vi "Insert_subvi_to_subpanel.vi"(5 "SubVI path":path, 6 "HART resource name":refnum<visa-resource-name>="HART", 7 "subpanel ref":refnum<vi>, 8 "Input number":i32, 9 "MODBUS resource name":refnum<visa-resource-name>="485", 10 "Index":u16(ring) items=["None", "Pulse Input", "Current Input", "Serial Input"], 11 "Array of VIs to insert":string[](array[string])) -> (0 "error out":errorcluster, 3 "VI reference out":refnum<vi>)   [LabVIEW 2016]
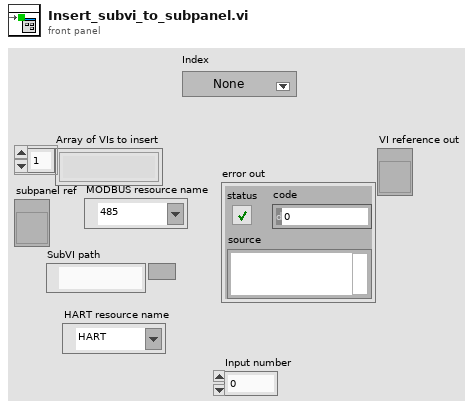
[diagram p1: front panel]
types:
  T1 = cluster{"Current Path":path, "DataFiles Path":path, "ReportFiles Path":path, "SupportFiles Path":path, "ReportTemplate Path":path, "Sample_pulses_VIT_Path":path, "Sample_current_VIT_Path":path, "Sample_MODBUS_VIT_Path":path}
  T2 = enum16{"Always On", "Always Off", "Off While Running"}
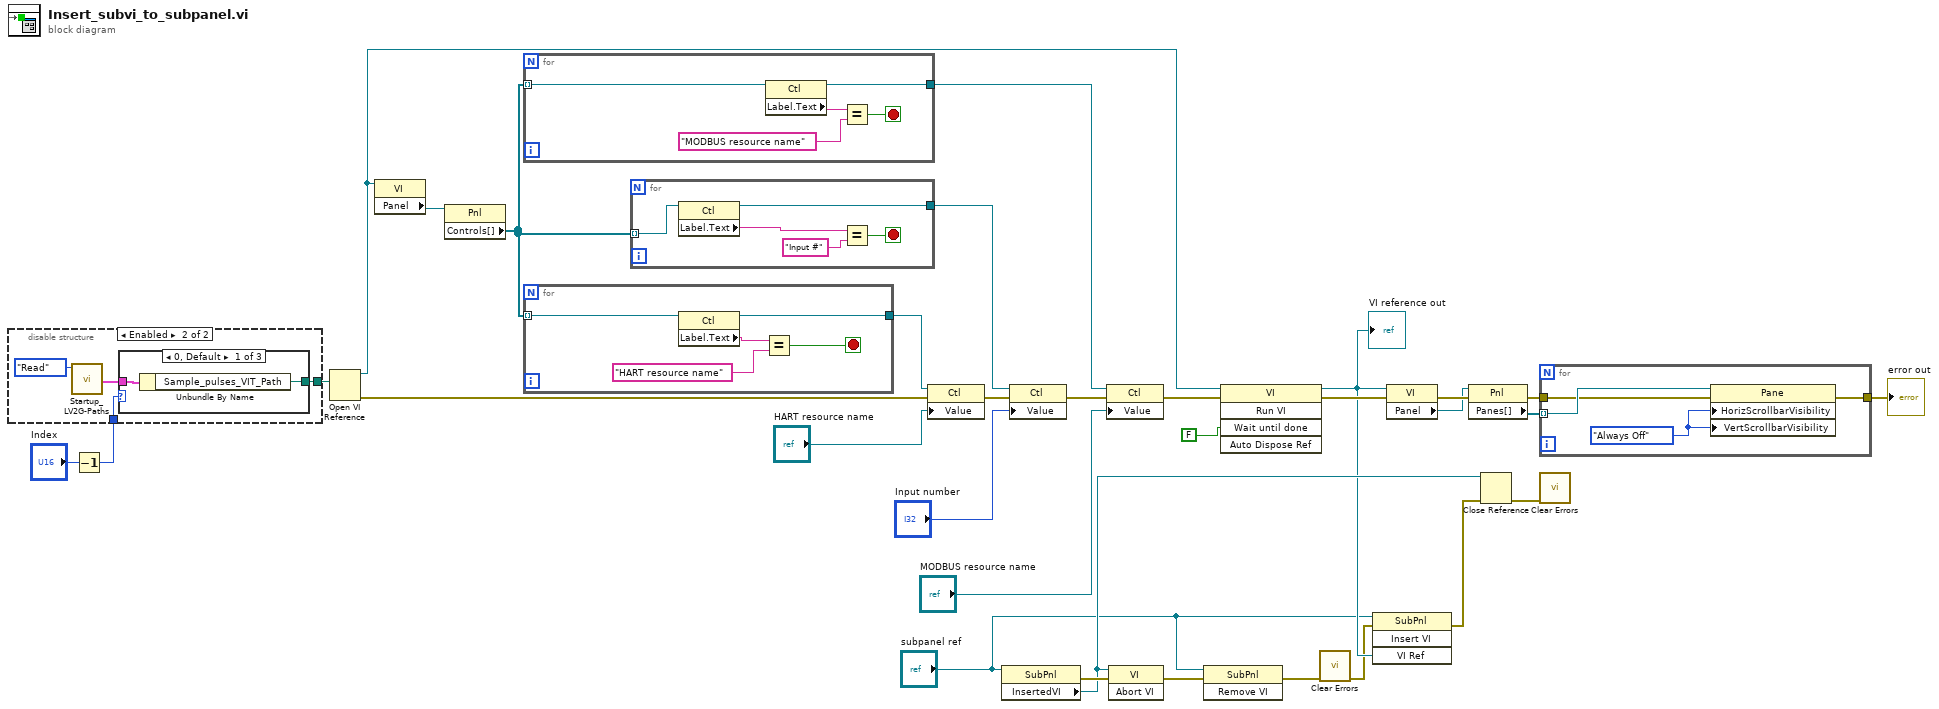
[diagram p0: block diagram]
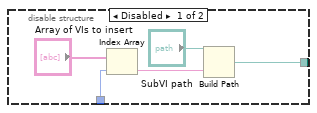
[diagram p2: hidden frame]
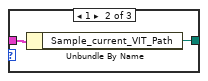
[diagram p3: hidden frame]
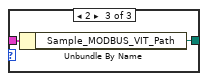
[diagram p4: hidden frame]
diagram:
  n1 = Decrement(x="Index") -> (x-1=w23:u16)
  n2 = disable-structure shown="Enabled" {
    disable-tunnel: [w37 w38] -> w30
    disable-tunnel: w23 -> [w35 w39]
    frame Disabled {
      n3 = Index Array(array="Array of VIs to insert", index=w35) -> (element=w36:string)
      n4 = Build Path(base path="SubVI path", name or relative path=w36) -> (appended path=w37:path)
    }
    frame Enabled {
      n5 = call "Startup_LV2G-Paths.vi"("Action"=enum16{"Read", "Write"}."Read") -> ("Paths"=w41:T1)  [unwired: 9 in, 1 out]
      n6 = case shown="0, Default" w39 {
        tunnel: w41 -> [w43 w45 w47]
        tunnel: [w42 w44 w46] -> w38
        frame 0, Default {
          n7 = Unbundle By Name(w43) -> ("Sample_pulses_VIT_Path"=w42:path)
        }
        frame 1 {
          n8 = Unbundle By Name(w45) -> ("Sample_current_VIT_Path"=w44:path)
        }
        frame 2 {
          n9 = Unbundle By Name(w47) -> ("Sample_MODBUS_VIT_Path"=w46:path)
        }
      }
    }
  }
  n10 = Open VI Reference(vi path=w30) -> (vi reference=w14:refnum<vi>, error out=w6:errorcluster)  [unwired: 5 in]
  n11 = property class="VI"(reference=w14) -> ("Panel"=w16:refnum<vi>)  [unwired: 1 in, 2 out]
  n12 = property class="Pnl"(reference=w16) -> ("Controls[]"=w4:refnum<vi>[])  [unwired: 1 in, 2 out]
  n13 = for {
    tunnel: w4 -> [w48] mode=indexing
    tunnel: [w49] -> w17
    stop <- w50 stop-if-true
    n14 = property class="Ctl"(reference=w48) -> (reference out=w49:refnum<vi>, "Label.Text"=w52:string)  [unwired: 1 in, 1 out]
    n15 = Equal?(x=w52, y="MODBUS resource name") -> (x = y?=w50:bool)
  }
  n16 = for {
    tunnel: w4 -> [w53] mode=indexing
    tunnel: [w54] -> w8
    stop <- w55 stop-if-true
    n17 = property class="Ctl"(reference=w53) -> (reference out=w54:refnum<vi>, "Label.Text"=w57:string)  [unwired: 1 in, 1 out]
    n18 = Equal?(x=w57, y="HART resource name") -> (x = y?=w55:bool)
  }
  n19 = for {
    tunnel: w4 -> [w58] mode=indexing
    tunnel: [w59] -> w5
    stop <- w60 stop-if-true
    n20 = property class="Ctl"(reference=w58) -> (reference out=w59:refnum<vi>, "Label.Text"=w62:string)  [unwired: 1 in, 1 out]
    n21 = Equal?(x=w62, y="Input #") -> (x = y?=w60:bool)
  }
  n22 = property class="Ctl"(reference=w8, error in=w6, "Value"="HART resource name") -> (error out=w3:errorcluster)  [unwired: 1 out]
  n23 = property class="SubPnl"(reference="subpanel ref") -> (error out=w29:errorcluster, "InsertedVI"=w27:refnum<vi>)  [unwired: 1 in, 1 out]
  n24 = property class="Ctl"(reference=w5, error in=w3, "Value"="Input number") -> (error out=w2:errorcluster)  [unwired: 1 out]
  n25 = property class="Ctl"(reference=w17, error in=w2, "Value"="MODBUS resource name") -> (error out=w15:errorcluster)  [unwired: 1 out]
  n26 = invoke class="VI" method="Abort VI"(reference=w27, error in=w29) -> (error out=w26:errorcluster)  [unwired: 1 in, 2 out]
  n27 = invoke class="SubPnl" method="Remove VI"(reference="subpanel ref", error in=w26) -> (error out=w25:errorcluster)  [unwired: 1 in, 2 out]
  n28 = invoke class="VI" method="Run VI"(reference=w14, error in=w15, "Wait until done"=FALSE ("Wait Until Done")) -> (reference out=w18:refnum<vi>, error out=w22:errorcluster)  [unwired: 2 in, 3 out]
  "VI reference out" <- w18
  n29 = call <vilib>:"Clear Errors.vi"("error in (no error)"=w25) -> ("error out"=w13:errorcluster)  [unwired: 5 in, 1 out]
  n30 = invoke class="SubPnl" method="Insert VI"(reference="subpanel ref", error in=w13, "VI Ref"=w18) -> (error out=w28:errorcluster)  [unwired: 1 in, 3 out]
  n31 = property class="VI"(reference=w18, error in=w22) -> (error out=w21:errorcluster, "Panel"=w19:refnum<vi>)  [unwired: 1 out]
  n32 = property class="Pnl"(reference=w19, error in=w21) -> (error out=w20:errorcluster, "Panes[]"=w32:refnum<vi>[])  [unwired: 1 out]
  n33 = Close Reference(reference=w27, error in (no error)=w28) -> (error out=w24:errorcluster)
  n34 = for {
    tunnel: w32 -> [w66] mode=indexing
    tunnel: w20 -> [w64]
    tunnel: [w63] -> w9
    w65 = T2."Always Off" ("Horizontal Scrollbar Visibility")
    n35 = property class="Pane"(reference=w66, error in=w64, "HorizScrollbarVisibility"=w65, "VertScrollbarVisibility"=w65) -> (error out=w63:errorcluster)  [unwired: 1 out]
  }
  "error out" <- w9
  n36 = call <vilib>:"Clear Errors.vi"("error in (no error)"=w24) -> ()  [unwired: 5 in, 2 out]
